vi "putIMSData.vi"(8 "error in (no error)":errorcluster, 10 "TelemetryIMSData":T1, 11 "M1M3SAL in":refnum<class "M1M3SAL.lvclass">) -> (0 "error out":errorcluster, 3 "M1M3SAL out":refnum<class "M1M3SAL.lvclass">)   [LabVIEW 2016, in "M1M3SupportCommunicator.lvlib" / "M1M3SAL.lvclass"]
uses:
  M1M3SAL.lvclass
  DataTypes/Topics/TelemetryIMSData.ctl
  DataTypes/Topics/Parts/Timestamp.ctl
  DataTypes/MessageHeader.ctl
  DataTypes/MessageTypes.ctl
  DataTypes/MessageTopics.ctl
  M1M3SAL.lvclass/M1M3SAL.ctl
  writeU8.vi
  writeI32.vi
  M1M3SupportCommunicator.lvlib
  DataTypes/Topics/M1M3SupportTopics.lvlib
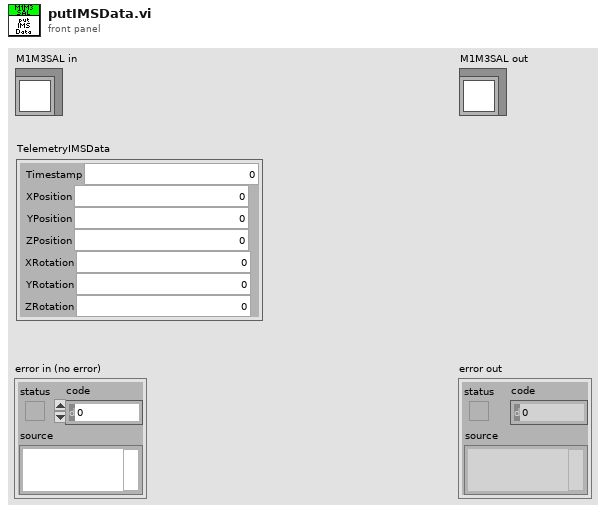
[diagram p1: front panel]
types:
  T1 = typedef "M1M3SupportTopics.lvlib/TelemetryIMSData.ctl" = cluster{"Timestamp":T2, "XPosition":dbl, "YPosition":dbl, "ZPosition":dbl, "XRotation":dbl, "YRotation":dbl, "ZRotation":dbl}
  T2 = typedef "M1M3SupportTopics.lvlib/Timestamp.ctl" = dbl
  T3 = typedef "M1M3SupportCommunicator.lvlib/MessageHeader.ctl" = cluster{"Type":T4, "Topic":T5, "Size":i32}
  T4 = typedef "M1M3SupportCommunicator.lvlib/MessageTypes.ctl" = enum8{"None", "PutSample", "GetNextSample", "LogEvent", "GetEvent", "IssueCommand", "CommandId", "WaitForCompletion", "AcceptCommand", "AckCommand"}
  T5 = typedef "M1M3SupportCommunicator.lvlib/MessageTopics.ctl" = enum8{"None", "ForceActuatorData", "MirrorForceData", "HardpointData", "AirData", "DynamicData", "FPGAData", "IMSData", "ForceActuatorStatus", "ElevationData", "HardpointStatus", "HardpointActuatorChase", "AirStatus", "ForceActuatorSafetyChecks", "ForceActuatorTest", "ActuatorBroadcastCounter", "StatusChecks", "CellChecks", "HardpointActuatorBreakaway", "RaiseMirrorComplete", "ILCCommunication", "ElevationAngleChecks", "DetailedState", "ServoLoops", "ForceActuatorInfo", "LowerMirrorComplete", "HardpointActuatorInfo", "SettingsApplied", "ErrorCode", "StartupChecks", "SummaryState", "SettingVersions", "ActuatorTestStatus", "AppliedSettingsMatchStart", "Enable", "EnterMaintenance", "Standby", "AbortLowerM1M3", "ApplyAberrationByForces", "ApplyAOSCorrectionByBendingModes", "ClearAOSCorrection", "Start", "RaiseM1M3", "TestForceActuator", "LowerM1M3", "ApplyAOSCorrectionByForces", "Disable", "ApplyAberationByBendingMode", "TestHardpoint", "ManipulateM1M3", "ClearAberration", "Exit", "TestAir", "AbortRaiseM1M3", "MoveHardpointActuators", "ExitMaintenance", "Shutdown"}
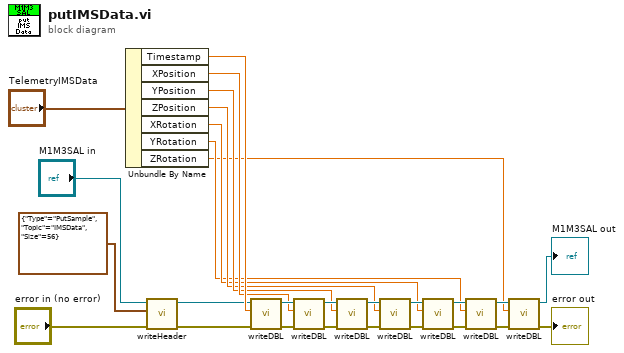
[diagram p0: block diagram]
diagram:
  n1 = Unbundle By Name("TelemetryIMSData") -> ("Timestamp"=w12:T2, "XPosition"=w11:dbl, "YPosition"=w10:dbl, "ZPosition"=w9:dbl, "XRotation"=w8:dbl, "YRotation"=w7:dbl, "ZRotation"=w6:dbl)
  n2 = call "writeHeader.vi"("error in (no error)"="error in (no error)", "MessageHeader"=T3 {"Type"=enum."PutSample", "Topic"=enum."IMSData", "Size"=56}, "M1M3SAL in"="M1M3SAL in") -> ("error out"=w2:errorcluster, "M1M3SAL out"=w3:refnum<class "M1M3SAL.lvclass">)  [unwired: 7 in]
  n3 = call "writeDBL.vi"("error in (no error)"=w2, "Input"=w12, "M1M3SAL in"=w3) -> ("error out"=w24:errorcluster, "M1M3SAL out"=w23:refnum<class "M1M3SAL.lvclass">)  [unwired: 7 in]
  n4 = call "writeDBL.vi"("error in (no error)"=w24, "Input"=w11, "M1M3SAL in"=w23) -> ("error out"=w22:errorcluster, "M1M3SAL out"=w21:refnum<class "M1M3SAL.lvclass">)  [unwired: 7 in]
  n5 = call "writeDBL.vi"("error in (no error)"=w22, "Input"=w10, "M1M3SAL in"=w21) -> ("error out"=w20:errorcluster, "M1M3SAL out"=w19:refnum<class "M1M3SAL.lvclass">)  [unwired: 7 in]
  n6 = call "writeDBL.vi"("error in (no error)"=w20, "Input"=w9, "M1M3SAL in"=w19) -> ("error out"=w18:errorcluster, "M1M3SAL out"=w17:refnum<class "M1M3SAL.lvclass">)  [unwired: 7 in]
  n7 = call "writeDBL.vi"("error in (no error)"=w18, "Input"=w8, "M1M3SAL in"=w17) -> ("error out"=w16:errorcluster, "M1M3SAL out"=w15:refnum<class "M1M3SAL.lvclass">)  [unwired: 7 in]
  n8 = call "writeDBL.vi"("error in (no error)"=w16, "Input"=w7, "M1M3SAL in"=w15) -> ("error out"=w14:errorcluster, "M1M3SAL out"=w13:refnum<class "M1M3SAL.lvclass">)  [unwired: 7 in]
  n9 = call "writeDBL.vi"("error in (no error)"=w14, "Input"=w6, "M1M3SAL in"=w13) -> ("error out"=→"error out":errorcluster, "M1M3SAL out"=→"M1M3SAL out":refnum<class "M1M3SAL.lvclass">)  [unwired: 7 in]
